vi "Add Connection to State.vi"(8 "error in":errorcluster, 9 "connection":T1, 10 "state":string, 11 "routing channel in":T2 format="%.0x") -> (0 "error out":errorcluster, 3 "routing channel out":T2=18446744073709551615 format="%.0x")   [LabVIEW 2020, in "Routing and Faulting Scripting.lvlib"]
doc: "Adds the connection to the state. The source and destination endpoints are connected when the state is active."
uses:
  Routing and Faulting Scripting.lvlib
  <vilib>/NI VeriStand/Custom Device API/Custom Device Item Ref.ctl
  Shared/Connection.ctl
  NationalInstruments.VeriStand.SystemDefinitionAPI
  Constants/Scripting Constants.vi
  <vilib>/NI VeriStand/Custom Device API/Custom Device API.lvlib
  Shared/Routing and Faulting Shared.lvlib
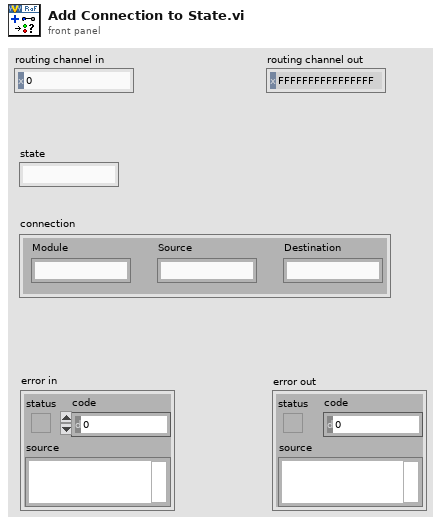
[diagram p1: front panel]
types:
  T1 = typedef "Routing and Faulting Shared.lvlib/Connection.ctl" = cluster{"Module":string, "Source":string, "Destination":string}
  T2 = typedef "Custom Device API.lvlib/Custom Device Item Ref.ctl" = u64
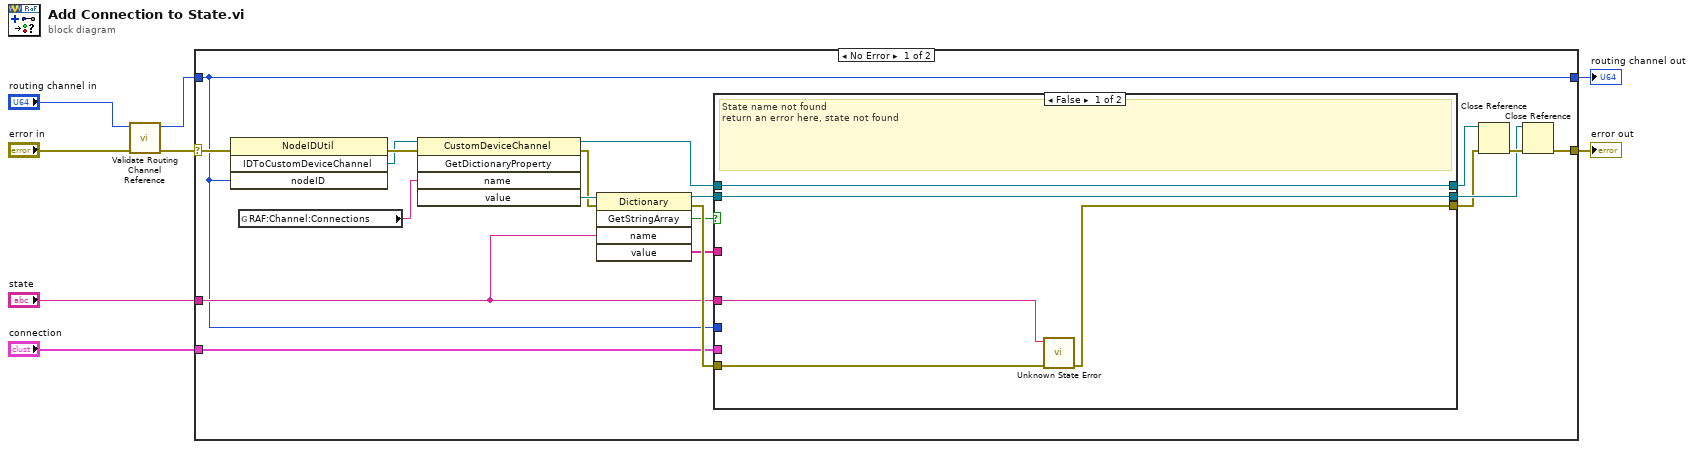
[diagram p0: block diagram]
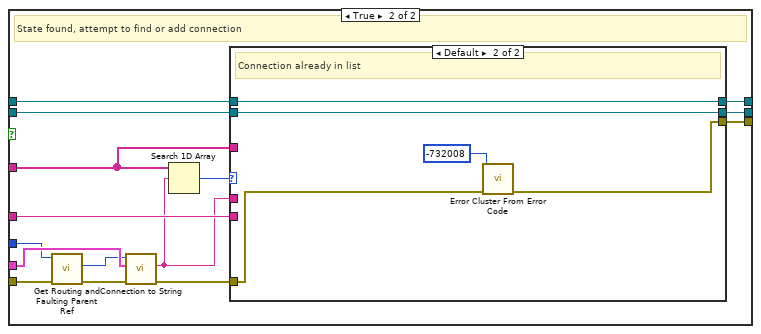
[diagram p2: hidden frame]
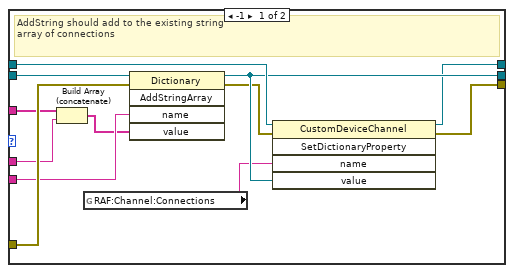
[diagram p3: hidden frame]
diagram:
  n1 = call "Validate Routing Channel Reference.vi"("error in"="error in", "routing channel in"="routing channel in") -> ("error out"=w3:errorcluster, "routing channel out"=w1:T2)  [unwired: 8 in]
  n2 = case shown="No Error" w3 {
    selector: w3 -> [w23 w66]
    tunnel: [w26 w66] -> w7
    tunnel: w1 -> [w9 w65]
    tunnel: [w9 w65] -> w6
    tunnel: "state" -> [w17 _]
    tunnel: "connection" -> [w12 _]
    frame No Error {
      n3 = invoke class="NodeIDUtil" method="IDToCustomDeviceChannel"(error in=w23, "nodeID"=w9) -> (error out=w24:errorcluster, "IDToCustomDeviceChannel"=w14:refnum<k24>)  [unwired: 2 in, 2 out]
      n4 = global read "Scripting Constants.vi" "RAF:Channel:Connections"() -> (w11:string)
      n5 = invoke class="CustomDeviceChannel" method="GetDictionaryProperty"(reference=w14, error in=w24, "name"=w11) -> (reference out=w10:refnum<k24>, error out=w20:errorcluster, "value"=w21:refnum<k24>)  [unwired: 2 in, 2 out]
      n6 = invoke class="Dictionary" method="GetStringArray"(reference=w21, error in=w20, "name"=w17) -> (reference out=w18:refnum<k24>, error out=w27:errorcluster, "GetStringArray"=w19:bool, "value"=w22:string[])  [unwired: 2 in, 1 out]
      n7 = case shown="False" w19 {
        tunnel: w22 -> [_ w40]
        tunnel: [w29 w46] -> w15
        tunnel: w17 -> [w28 w45]
        tunnel: w18 -> [w32 w44]
        tunnel: [w32 w43] -> w16
        tunnel: w10 -> [w31 w42]
        tunnel: [w31 w41] -> w13
        tunnel: w12 -> [_ w39]
        tunnel: w9 -> [_ w36]
        tunnel: w27 -> [w30 w35]
        frame False {
          # "State name not found\nreturn an error here, state not found"
          n8 = call "Unknown State Error.vi"("error in (no error)"=w30, "state"=w28) -> ("error out"=w29:errorcluster)  [unwired: 9 in]
        }
        frame True {
          # "State found, attempt to find or add connection"
          n9 = call "Get Routing and Faulting Parent Ref.vi"("error in"=w35, "routing and faulting child in"=w36) -> ("error out"=w34:errorcluster, "routing and faulting"=w33:T2)  [unwired: 7 in, 1 out]
          n10 = call "Connection to String.vi"("error in"=w34, "connection"=w39, "routing and faulting in"=w33) -> ("error out"=w37:errorcluster, "string"=w38:string)  [unwired: 5 in, 2 out]
          n11 = Search 1D Array(1D array=w40, element=w38) -> (index of element=w47:i32)  [unwired: 1 in]
          n12 = case shown="Default" w47 {
            tunnel: [w53 w63] -> w46
            tunnel: w45 -> [w58 _]
            tunnel: w44 -> [w57 w62]
            tunnel: [w55 w62] -> w43
            tunnel: w42 -> [w56 w61]
            tunnel: [w52 w61] -> w41
            tunnel: w40 -> [w51 _]
            tunnel: w38 -> [w50 _]
            tunnel: w37 -> [w59 w60]
            frame -1 {
              # "AddString should add to the existing string\narray of connections"
              n13 = Build Array (concatenate)(w51, w50) -> (w49:string[])
              n14 = global read "Scripting Constants.vi" "RAF:Channel:Connections"() -> (w48:string)
              n15 = invoke class="Dictionary" method="AddStringArray"(reference=w57, error in=w59, "name"=w58, "value"=w49) -> (reference out=w55:refnum<k24>, error out=w54:errorcluster)  [unwired: 1 in, 3 out]
              n16 = invoke class="CustomDeviceChannel" method="SetDictionaryProperty"(reference=w56, error in=w54, "name"=w48, "value"=w55) -> (reference out=w52:refnum<k24>, error out=w53:errorcluster)  [unwired: 1 in, 3 out]
            }
            frame Default {
              # "Connection already in list"
              n17 = call <vilib>:"Error Cluster From Error Code.vi"("error in (no error)"=w60, "error code (0)"=-732008) -> ("error out"=w63:errorcluster)  [unwired: 7 in]
            }
          }
        }
      }
      n18 = Close Reference(reference=w13, error in (no error)=w15) -> (error out=w25:errorcluster)
      n19 = Close Reference(reference=w16, error in (no error)=w25) -> (error out=w26:errorcluster)
    }
    frame Error {
    }
  }
  "routing channel out" <- w6
  "error out" <- w7
